vi "ApplicationInfos.vi"(8 "error in (no error)":errorcluster) -> (0 "error out":errorcluster, 3 "ApplicationInfo":T1)   [LabVIEW 2013]
uses:
  ApplicationInfos.ctl
panel:
  # "Informations \ngénérales de\nl'application"
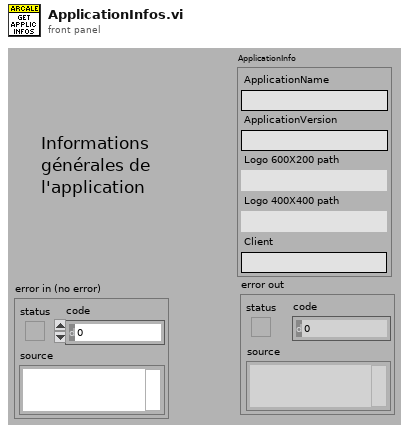
[diagram p1: front panel]
types:
  T1 = typedef "ApplicationInfos.ctl" = cluster{"ApplicationName":string, "ApplicationVersion":string, "Logo 600X200 path":path, "Logo 400X400 path":path, "Client":string}
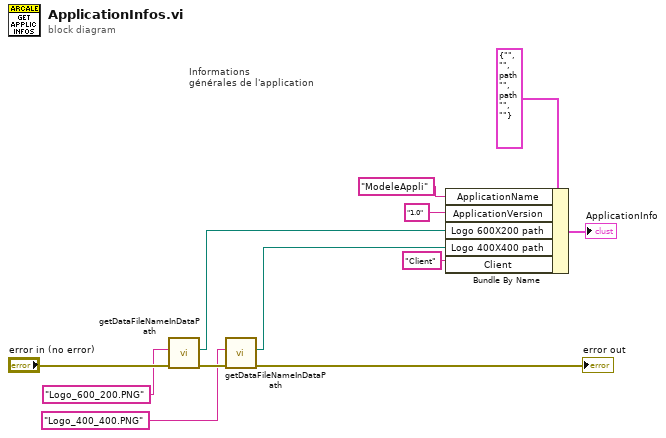
[diagram p0: block diagram]
diagram:
  # "Informations \ngénérales de l'application"
  n1 = call "getDataFileNameInDataPath.vi"("error in (no error)"="error in (no error)", "FileName"="Logo_600_200.PNG") -> ("error out"=w11:errorcluster, "FileNamePathInDataDir"=w7:path)  [unwired: 8 in]
  n2 = call "getDataFileNameInDataPath.vi"("error in (no error)"=w11, "FileName"="Logo_400_400.PNG") -> ("error out"=→"error out":errorcluster, "FileNamePathInDataDir"=w1:path)  [unwired: 8 in]
  n3 = Bundle By Name(cluster=T1 {"ApplicationName"="", "ApplicationVersion"="", "Logo 600X200 path"=path "", "Logo 400X400 path"=path "", "Client"=""} ("ApplicationInfo"), "ApplicationName"="ModeleAppli", "ApplicationVersion"="1.0" ("ApplicationName"), "Logo 600X200 path"=w7, "Logo 400X400 path"=w1, "Client"="Client") -> (→"ApplicationInfo":T1)
